vi "Format Error.vi"(9 "Call Chain":string[](array[string]), 10 "Error To Log":errorcluster, 11 "IErrorFormat in":refnum<class "IErrorFormat.lvclass">) -> (3 "Error String":string)   [LabVIEW 2020, in "MVA Framework.lvlib" / "Composed Log.lvlib" / "IErrorFormat.lvclass"]
uses:
  IErrorFormat.lvclass
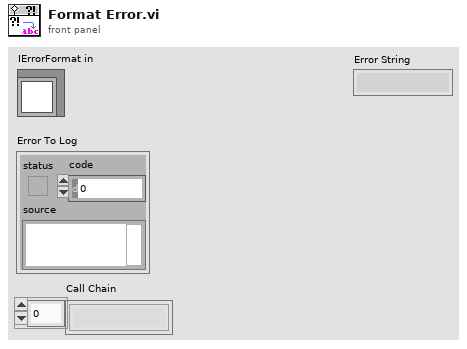
[diagram p1: front panel]
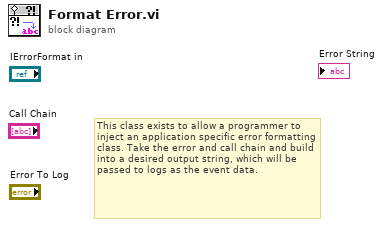
[diagram p0: block diagram]
diagram:
  # "This class exists to allow a programmer to inject an application specific error formatting class. Take the error and call chain and build into a desired output string, which will be passed to logs as the event data."
